vi "Get Array Fundamental Type.vi"(9 "error in (no error)":errorcluster, 10 ".NET AdsDataType":refnum<k24>) -> (1 "error out":errorcluster, 2 "Fundametal .NET AdsDataType":refnum<k24>, 3 "Fundamental PLC Type":T1, 5 "Dimension Lengths":i32[](array[numeric]))   [LabVIEW 2018, in "TwinCAT ADS.lvclass"]
uses:
  TwinCAT ADS.lvclass
  TwinCAT.Ads
  Controls/PLC Type.ctl
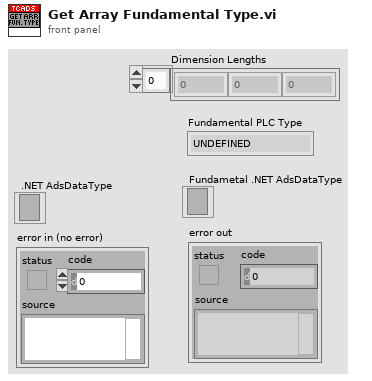
[diagram p1: front panel]
types:
  T1 = typedef "TwinCAT ADS.lvclass/PLC Type.ctl" = enum16{"UNDEFINED", "INT", "DINT", "REAL", "LREAL", "SINT", "BYTE", "UINT", "UDINT", "LINT", "ULINT", "STRING", "WSTRING", "BOOL", "TIME", "LTIME", "DATE", "DT", "TOD", "ARRAY", "JAGGED ARRAY", "STRUCT", "FUNCTION BLOCK", "UNION", "POINTER", "USER DEFINED"}
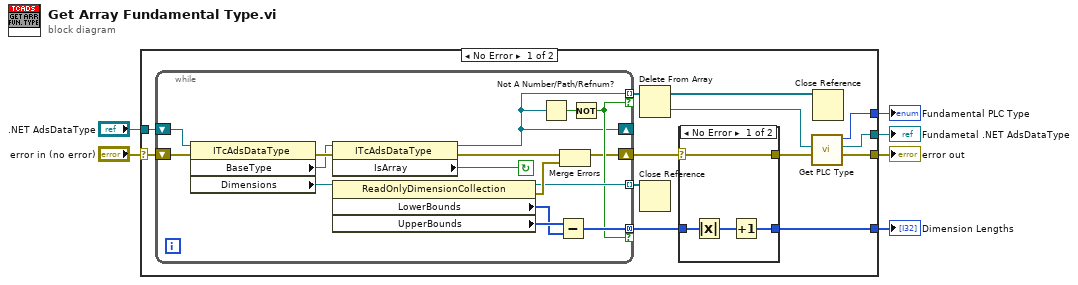
[diagram p0: block diagram]
diagram:
  n1 = case shown="No Error" "error in (no error)" {
    selector: "error in (no error)" -> [w7 w41]
    tunnel: ".NET AdsDataType" -> [w15 _]
    tunnel: [w14 w41] -> w5
    tunnel: [w12 _] -> w4
    tunnel: [w11 _] -> w3
    tunnel: [w10 _] -> w2
    frame No Error {
      n2 = while {
        shift-right: [w26] -> w9
        shift-left: w7 -> [w39]
        shift-right: [w29] -> _
        shift-left: w15 -> [w38]
        tunnel: [w37] -> w13 mode=concatenating if=w32
        tunnel: [w29] -> w18 mode=indexing if=w32
        tunnel: [w33] -> w19 mode=indexing
        stop <- w25 continue-if-true
        n3 = property class="ITcAdsDataType"(reference=w38, error in=w39) -> (error out=w30:errorcluster, "BaseType"=w28:refnum<k24>, "Dimensions"=w31:refnum<k24>)  [unwired: 1 out]
        n4 = property class="ITcAdsDataType"(reference=w28, error in=w30) -> (reference out=w29:refnum<k24>, error out=w27:errorcluster, "IsArray"=w25:bool)
        n5 = property class="ReadOnlyDimensionCollection"(reference=w31) -> (reference out=w33:refnum<k24>, error out=w40:errorcluster, "LowerBounds"=w35:i32[], "UpperBounds"=w36:i32[])  [unwired: 1 in]
        n6 = Not A Number/Path/Refnum?(number/path/refnum=w29) -> (NaN/Path/Refnum?=w34:bool)
        n7 = Subtract(x=w36, y=w35) -> (x-y=w37:i32[])
        n8 = Merge Errors(w27, w40) -> (w26:errorcluster)
        n9 = Not(x=w34) -> (.not. x?=w32:bool)
      }
      n10 = Delete From Array(array=w18) -> (deleted portion=w16:refnum<k24>, array with subset deleted=w17:refnum<k24>[])  [unwired: 2 in]
      n11 = Close Reference(reference=w19) -> ()  [unwired: 1 in, 1 out]
      n12 = case shown="No Error" w9 {
        selector: w9 -> [w21 w24]
        tunnel: w13 -> [w23 _]
        tunnel: [w22 _] -> w10
        tunnel: [w21 w24] -> w8
        frame No Error {
          n13 = Absolute Value(x=w23) -> (abs(x)=w20:i32[])
          n14 = Increment(x=w20) -> (x+1=w22:i32[])
        }
        frame Error {
        }
      }
      n15 = call "Get PLC Type.vi"("error in (no error)"=w8, ".NET AdsDataType in"=w16) -> ("error out"=w14:errorcluster, ".NET AdsDataType"=w12:refnum<k24>, "PLC Type"=w11:T1)  [unwired: 7 in]
      n16 = Close Reference(reference=w17) -> ()  [unwired: 1 in, 1 out]
    }
    frame Error {
    }
  }
  "error out" <- w5
  "Fundamental PLC Type" <- w3
  "Fundametal .NET AdsDataType" <- w4
  "Dimension Lengths" <- w2
